vi "ge_GetTagContents.vi"(6 "String ID":string, 7 "Array Container?":bool, 8 "error in":errorcluster, 9 "Item XML":string, 10 "Array Attributes":string, 11 "Item Name/Type":cluster{"Type Enum":T1, "Item Name":string}) -> (0 "error out":errorcluster, 1 "XML After Closing Tag":string, 3 "Item XML Data":T2)   [LabVIEW 2012]
uses:
  <vilib>/Utility/VariantDataType/Type.ctl
  <vilib>/regexp/Match Regular Expression.xnode
  <vilib>/Utility/VariantDataType/VariantType.lvlib
panel:
  out "whole match":string
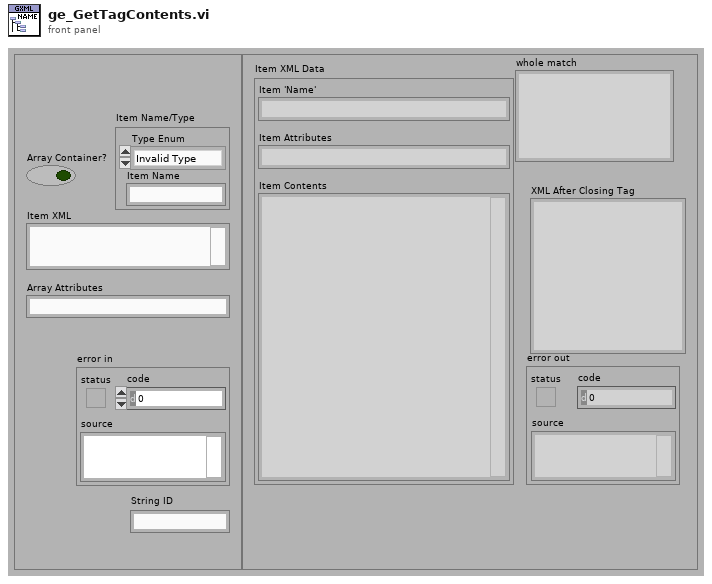
[diagram p1: front panel]
types:
  T1 = typedef "VariantType.lvlib/Type.ctl" = enum8{"Invalid Type", "Void", "I8", "I16", "I32", "I64", "U8", "U16", "U32", "U64", "Single Float", "Double Float", "Extended Float", "Single Complex", "Double Complex", "Extended Complex", "Enum U8", "Enum U16", "Enum U32", "Enum U64", "Single Float With Unit", "Double Float With Unit", "Extended Float With Unit", "Single Complex with Unit", "Double Complex with Unit", "Extended Complex with Unit", "Boolean", "String", "Path", "Picture", "Tag", "Array", "Cluster", "Variant", "LV Variant", "Waveform", "Timestamp", "Digital Waveform", "Digital Data", "ExpressData", "Refnum", "External Data", "VI", "Poly VI", "LabVIEW Class Instance", "Fixed Point"}
  T2 = cluster{"Item 'Name'":string, "Item Attributes":string, "Item Contents":string}
  T3 = cluster{"XML String":string, "XML String":string, "XML String":string}
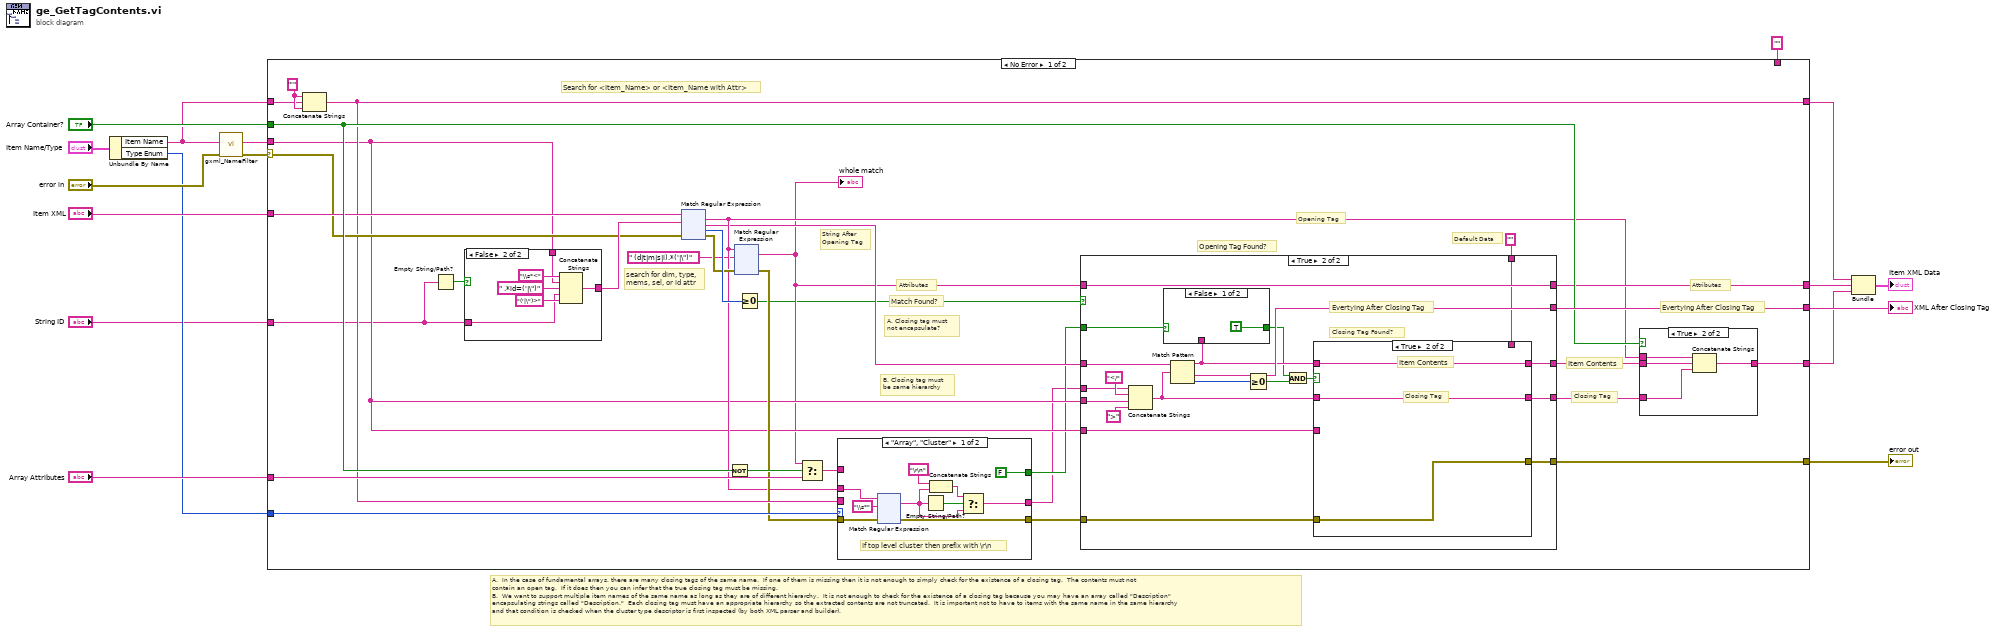
[diagram p0: block diagram]
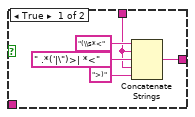
[diagram p2: hidden frame]
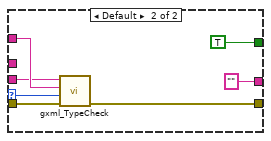
[diagram p3: hidden frame]
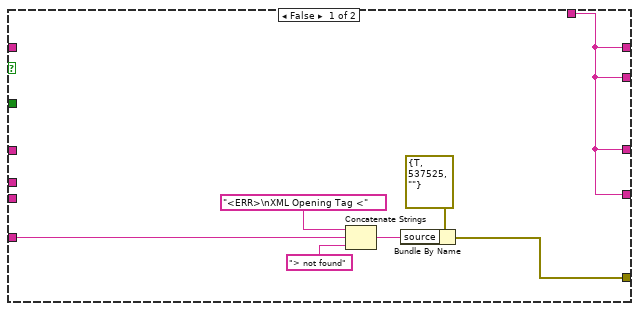
[diagram p5: hidden frame]
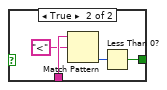
[diagram p6: hidden frame]
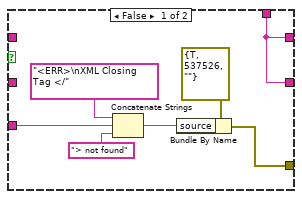
[diagram p7: hidden frame]
diagram:
  # "A.  In the case of fundamental arrays, there are many closing tags of the same name.  If one of them is missing then it is not enough to simply check for the existence of a closing tag.  The contents must not\ncontain an open tag.  If it does then you can infer that the true closing tag must be missing.\nB.  We want to support multiple item names of the same name as long as they are of different hierarchy.  It is not enough to check for the existence of a closing tag because you may have an array called \"Description\"\nencapsulating strings called \"Description.\"  Each closing tag must have an appropriate hierarchy so the extracted contents are not truncated.  It is important not to have to items with the same name in the same hierarchy\nand that condition is checked when the cluster type descriptor is first inspected (by both XML parser and builder)."
  n1 = Unbundle By Name("Item Name/Type") -> ("Item Name"=w5:string, "Type Enum"=w2:T1)
  n2 = call <userlib>:"gxml_NameFilter.vi"("error in"="error in", "Tag Name"=w5) -> ("error out"=w11:errorcluster, "Tag_Name"=w10:string)  [unwired: 7 in]
  n3 = case shown="No Error" w11 {
    selector: w11 -> [w35 w459]
    tunnel: w10 -> [w25 _]
    tunnel: [w48 w458] -> w8
    tunnel: [w42 w458] -> w9
    tunnel: "Item XML" -> [w39 _]
    tunnel: [w32 w459] -> w16
    tunnel: [w49 w458] -> w15
    tunnel: "Array Container?" -> [w43 _]
    tunnel: "Array Attributes" -> [w45 _]
    tunnel: w5 -> [w33 _]
    tunnel: [w30 w458] -> w3
    tunnel: "" ("XML String") -> [_ w458]
    tunnel: w2 -> [w31 _]
    tunnel: "String ID" -> [w18 _]
    frame No Error {
      w34 = "'" ("string")
      # "A. Closing tag must\nnot encapsulate?"
      # "search for dim, type,\nmems, sel, or id attr"
      # "Closing Tag"
      # "B. Closing tag must\nbe same hierarchy"
      # "Match Found?"
      # "Attributes"
      # "Search for <Item_Name> or <Item_Name with Attr>"
      # "String After\nOpening Tag"
      # "Evertying After Closing Tag"
      # "Item Contents"
      # "Opening Tag"
      # "Attributes"
      # "Opening Tag Found?"
      # "Default Data"
      n4 = Concatenate Strings(w34, w33, w34) -> (w30:string)
      n5 = Empty String/Path?(string/path=w18) -> (empty?=w19:bool)
      n6 = case shown="False" w19 {
        tunnel: [w52 w59] -> w37
        tunnel: w25 -> [w50 w58]
        tunnel: w18 -> [_ w55]
        frame True {
          n7 = Concatenate Strings("(\\s*<", w50, " .*('|\")>| *<" ("regular expression"), w50, ">)" ("regular expression")) -> (w52:string)
        }
        frame False {
          n8 = Concatenate Strings("\\s*<", w58, " .*id=('|\")" ("regular expression"), w55, "('|\")>" ("regular expression")) -> (w59:string)
        }
      }
      n9 = xnode "Match Regular Expression"("input string"=w39, "regular expression"=w37, "error in"=w35) -> ("whole match"=w27:string, "after match"=w24:string, "offset past match"=w38:i32, "error out"=w36:errorcluster)  [unwired: 3 in, 1 out]
      n10 = Not(x=w43) -> (.not. x?=w44:bool)
      n11 = xnode "Match Regular Expression"("input string"=w27, "regular expression"=" (d|t|m|s|i).*('|\")", "error in"=w36) -> ("whole match"=w21:string, "error out"=w28:errorcluster)  [unwired: 3 in, 3 out]
      "whole match" <- w21
      n12 = Greater Or Equal To 0?(x=w38) -> (x >= 0?=w20:bool)
      n13 = Select(t=w21, s=w44, f=w45) -> (s? t:f=w46:string)
      n14 = case shown="\"Array\", \"Cluster\"" w31 {
        selector: w31 -> [_ w406]
        tunnel: w46 -> [_ w410]
        tunnel: [w290 w409] -> w41
        tunnel: w28 -> [w291 w407]
        tunnel: w30 -> [_ w408]
        tunnel: w27 -> [w289 _]
        tunnel: [w286 "" ("whole match")] -> w22
        tunnel: [FALSE TRUE] -> w23
        frame "Array", "Cluster" {
          # "If top level cluster then prefix with \\r\\n"
          n15 = xnode "Match Regular Expression"("input string"=w289, "regular expression"="\\s*", "error in"=w291) -> ("whole match"=w287:string, "error out"=w290:errorcluster)  [unwired: 3 in, 3 out]
          n16 = Empty String/Path?(string/path=w287) -> (empty?=w285:bool)
          n17 = Concatenate Strings("\r\n" ("string"), w287) -> (w283:string)
          n18 = Select(t=w283, s=w285, f=w287) -> (s? t:f=w286:string)
        }
        frame Default {
          n19 = call <userlib>:"gxml_TypeCheck.vi"("error in"=w407, "Type Enum"=w406, "XML Item Attributes"=w410, "Item Name"=w408) -> ("error out"=w409:errorcluster)  [unwired: 7 in]
        }
      }
      n20 = case shown="True" w20 {
        tunnel: [w416 w442] -> w40
        tunnel: w25 -> [w419 w440]
        tunnel: [w418 w441] -> w32
        tunnel: w21 -> [_ w438]
        tunnel: [w416 w438] -> w42
        tunnel: [w416 w437] -> w49
        tunnel: w41 -> [_ w436]
        tunnel: "" ("XML String") -> [w416 w435]
        tunnel: [w416 w434] -> w29
        tunnel: w22 -> [_ w430]
        tunnel: w25 -> [_ w429]
        tunnel: w24 -> [_ w428]
        tunnel: w23 -> [_ w426]
        frame False {
          n21 = Concatenate Strings("<ERR>\nXML Opening Tag <" ("string"), w419, "> not found") -> (w421:string)
          n22 = Bundle By Name(cluster=errorcluster {"status"=TRUE, "code"=537525, "source"=""} ("error IO"), "source"=w421) -> (w418:errorcluster)
        }
        frame True {
          # "Evertying After Closing Tag"
          # "Closing Tag Found?"
          n23 = Concatenate Strings(w430, "</", w429, ">" ("string")) -> (w431:string)
          n24 = Match Pattern(string=w428, regular expression=w431) -> (before substring=w427:string, after substring=w437:string, offset past match=w439:i32)  [unwired: 1 in, 1 out]
          n25 = case shown="False" w426 {
            tunnel: w427 -> [_ w447]
            tunnel: [TRUE w444] -> w424
            frame False {
            }
            frame True {
              n26 = Match Pattern(string=w447, regular expression="<") -> (offset past match=w445:i32)  [unwired: 1 in, 3 out]
              n27 = Less Than 0?(x=w445) -> (x < 0?=w444:bool)
            }
          }
          n28 = Greater Or Equal To 0?(x=w439) -> (x >= 0?=w425:bool)
          n29 = And(x=w424, y=w425) -> (x .and. y?=w423:bool)
          n30 = case shown="True" w423 {
            tunnel: w427 -> [_ w457]
            tunnel: [w448 w457] -> w442
            tunnel: [w451 w456] -> w441
            tunnel: w440 -> [w450 _]
            tunnel: w436 -> [_ w456]
            tunnel: w435 -> [w448 _]
            tunnel: w431 -> [_ w455]
            tunnel: [w448 w455] -> w434
            frame False {
              n31 = Concatenate Strings("<ERR>\nXML Closing Tag </" ("string"), w450, "> not found") -> (w453:string)
              n32 = Bundle By Name(cluster=errorcluster {"status"=TRUE, "code"=537526, "source"=""} ("error IO"), "source"=w453) -> (w451:errorcluster)
            }
            frame True {
              # "Closing Tag"
              # "Item Contents"
            }
          }
        }
      }
      n33 = case shown="True" w43 {
        tunnel: w40 -> [w411 w415]
        tunnel: [w411 w414] -> w48
        tunnel: w27 -> [_ w413]
        tunnel: w29 -> [_ w412]
        frame False {
        }
        frame True {
          n34 = Concatenate Strings(w413, w415, w412) -> (w414:string)
        }
      }
    }
    frame Error {
    }
  }
  "error out" <- w16
  "XML After Closing Tag" <- w15
  n35 = Bundle("XML String"=w3, "XML String"=w9, "XML String"=w8) -> (→"Item XML Data":T3)  [unwired: 1 in]
